vi "resetLockout.vi"(8 "error in":errorcluster, 9 "Boiler Simulation Controls":refnum<vi>, 10 "Boiler Controls":refnum<vi>, 11 "Boiler Status Indicators":refnum<vi>) -> (0 "error out":errorcluster, 3 "Ready?":bool)   [LabVIEW 2024]
uses:
  Controls/Boiler Simulation Controls.ctl
  Controls/Boiler Status Indicators.ctl
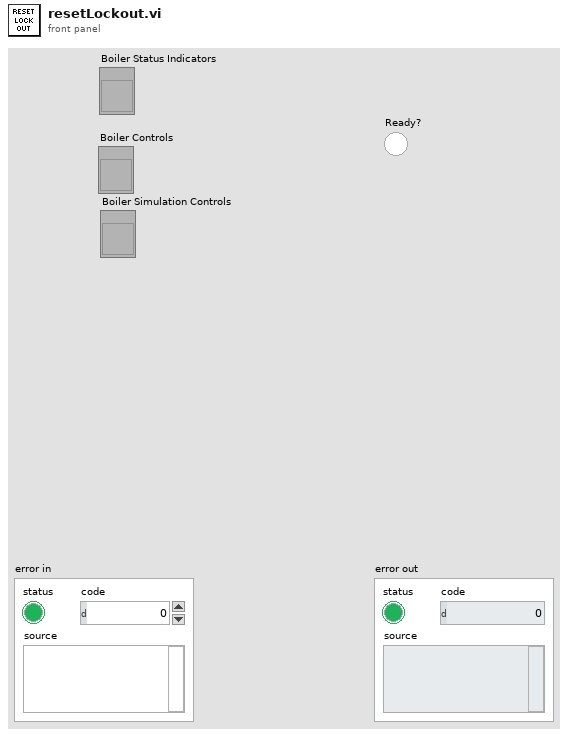
[diagram p1: front panel]
types:
  T1 = typedef "Boiler Simulation Controls.ctl" = cluster{"Flame Sensor Value (%)":dbl, "Run Interlock":bool, "Forced Draft Fan":bool}
  T2 = typedef "Boiler Controls.ctl" = cluster{"Boiler Reset":bool, "Start Sequence":bool, "Pilot":bool, "Shutdown":bool, "Fuel Valve Position":dbl}
  T3 = typedef "Boiler Status Indicators.ctl" = cluster{"Status":string, "Primary Fan":bool, "Natural Gas Valve":bool, "Pilot":bool, "Fuel Valve":bool, "Forced Draft Fan":bool, "Time Count":dbl}
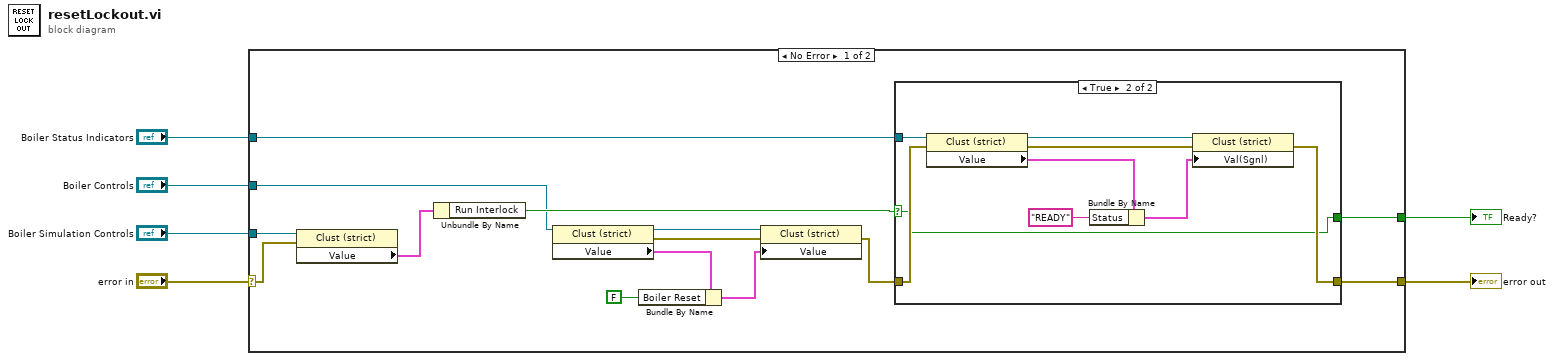
[diagram p0: block diagram]
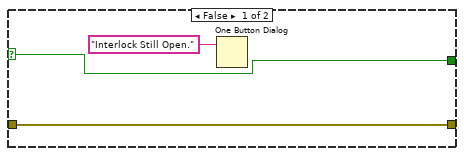
[diagram p2: hidden frame]
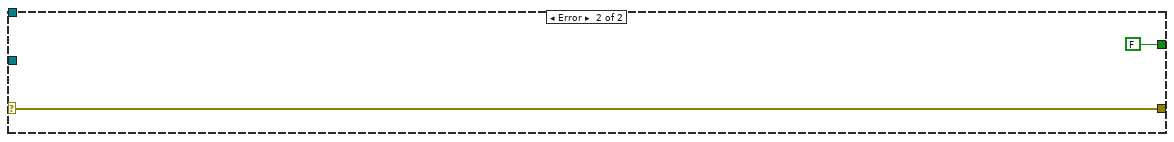
[diagram p3: hidden frame]
diagram:
  n1 = case shown="No Error" "error in" {
    selector: "error in" -> [w19 w34]
    tunnel: [w16 w34] -> w5
    tunnel: "Boiler Simulation Controls" -> [w20 _]
    tunnel: "Boiler Status Indicators" -> [w15 _]
    tunnel: [w14 FALSE] -> w2
    tunnel: "Boiler Controls" -> [w13 _]
    frame No Error {
      n2 = property class="Clust (strict)"(reference=w20, error in=w19) -> ("Value"=w18:T1)  [unwired: 2 out]
      n3 = Unbundle By Name(w18) -> ("Run Interlock"=w17:bool)
      n4 = property class="Clust (strict)"(reference=w13) -> (reference out=w12:refnum<vi>, error out=w11:errorcluster, "Value"=w9:T2)  [unwired: 1 in]
      n5 = Bundle By Name(cluster=w9, "Boiler Reset"=FALSE) -> (w8:T2)
      n6 = property class="Clust (strict)"(reference=w12, error in=w11, "Value"=w8) -> (error out=w10:errorcluster)  [unwired: 1 out]
      n7 = case shown="True" w17 {
        selector: w17 -> [w21 w24]
        tunnel: [w22 w25] -> w16
        tunnel: w10 -> [w22 w27]
        tunnel: w15 -> [_ w32]
        tunnel: [w21 w24] -> w14
        frame False {
          n8 = One Button Dialog(message="Interlock Still Open.") -> ()  [unwired: 1 in, 1 out]
        }
        frame True {
          n9 = property class="Clust (strict)"(reference=w32, error in=w27) -> (reference out=w31:refnum<vi>, error out=w26:errorcluster, "Value"=w30:T3)
          n10 = Bundle By Name(cluster=w30, "Status"="READY") -> (w29:T3)
          n11 = property class="Clust (strict)"(reference=w31, error in=w26, "Val(Sgnl)"=w29) -> (error out=w25:errorcluster)  [unwired: 1 out]
        }
      }
    }
    frame Error {
    }
  }
  "error out" <- w5
  "Ready?" <- w2
